vi "getMagnetVector.vi"(8 "error in (no error)":errorcluster, 11 "Instrument.Cryostat in":refnum<class "Instrument.Cryostat.lvclass">) -> (0 "error out":errorcluster, 1 "Status":string, 2 "Field (T)":dbl[](array[numeric]), 3 "Instrument.Cryostat out":refnum<class "Instrument.Cryostat.lvclass">, 4 "Finished?":bool)   [LabVIEW 2019, in "Instrument.Cryostat.lvclass"]
uses:
  Instrument.Cryostat.lvclass
  Typedefs/getMagnetVector--cluster.ctl
  Typedefs/Cryostat.commands--enum.ctl
  467153f6-b5b3-463b-bb65-50ad0ef35abd.vi
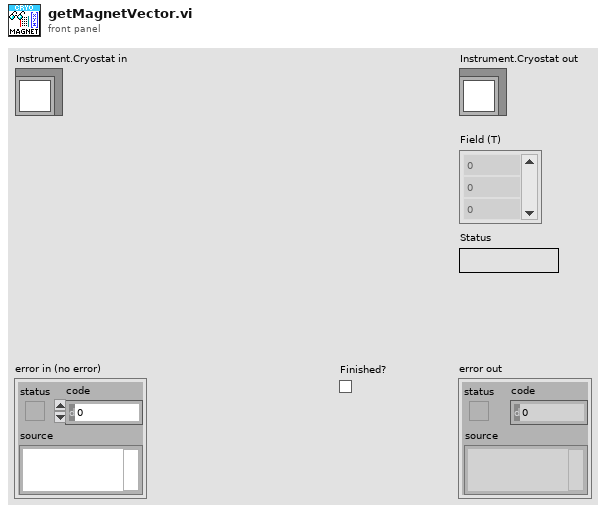
[diagram p1: front panel]
types:
  T1 = typedef "Instrument.Cryostat.lvclass/Cryostat.commands--enum.ctl" = enum16{"getLN2Level", "getLHeLevel", "getMagnet", "getMagnetVector", "setMagnet", "setMagnetVector", "getAngle", "setAngle", "getTemperature", "setTemperature", "getHeater", "setHeater", "getChamber", "setChamber", "getPressure"}
  T2 = typedef "Instrument.Cryostat.lvclass/getMagnetVector--cluster.ctl" = cluster{"field":dbl[], "status":string, "finished":bool}
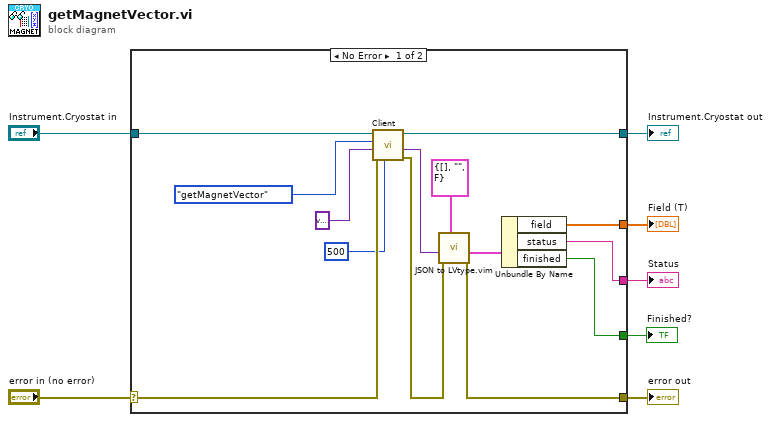
[diagram p0: block diagram]
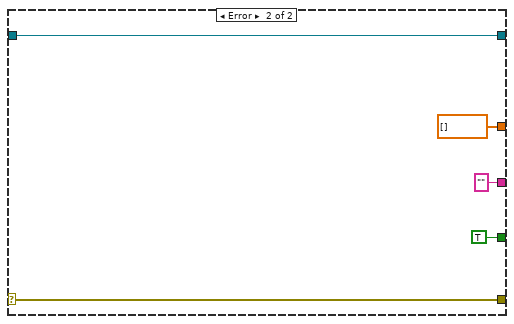
[diagram p2: hidden frame]
diagram:
  n1 = case shown="No Error" "error in (no error)" {
    selector: "error in (no error)" -> [w15 w26]
    tunnel: [w12 w26] -> w6
    tunnel: [w21 w25] -> w4
    tunnel: "Instrument.Cryostat in" -> [w16 w25]
    tunnel: [w20 dbl[] [] ("Field (T)")] -> w3
    tunnel: [w19 "" ("Status")] -> w2
    tunnel: [w18 TRUE] -> w1
    frame No Error {
      n2 = call-dynamic "Client.vi"("timeout (ms) [500]"=500, "error in (no error)"=w15, "Data in"=variant, "Command in"=Cryostat.commands--enum."getMagnetVector" ("commands"), "Instrument in"=w16) -> ("error out"=w13:errorcluster, "Data out"=w14:variant, "Instrument out"=w21:refnum<class "Instrument.Cryostat.lvclass">)  [unwired: 3 in, 1 out]
      n3 = call "JSON to LVtype.vim"("type"=T2 {"field"=[], "status"="", "finished"=FALSE} ("getMagnet"), "error in (no error)"=w13, "JSON Data in"=w14) -> ("error out"=w12:errorcluster, "Data out"=w11:T2)  [unwired: 7 in]
      n4 = Unbundle By Name(w11) -> ("field"=w20:dbl[], "status"=w19:string, "finished"=w18:bool)
    }
    frame Error {
    }
  }
  "error out" <- w6
  "Instrument.Cryostat out" <- w4
  "Field (T)" <- w3
  "Status" <- w2
  "Finished?" <- w1
